vi "Import VeriStand Mappings.vi"() -> ()   [LabVIEW 2016]
uses:
  NationalInstruments.VeriStand.SystemDefinitionAPI
  <vilib>/Utility/file.llb/Read Delimited Spreadsheet (string).vi
panel:
  out "String":string="Running..."
  in  "System Definition File (.nivssdf)":path
  in  "System Mappings File (.txt)":path
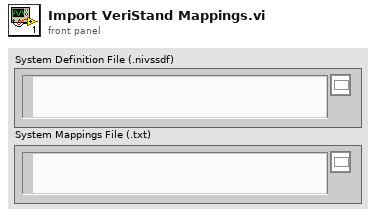
[diagram p1: front panel]
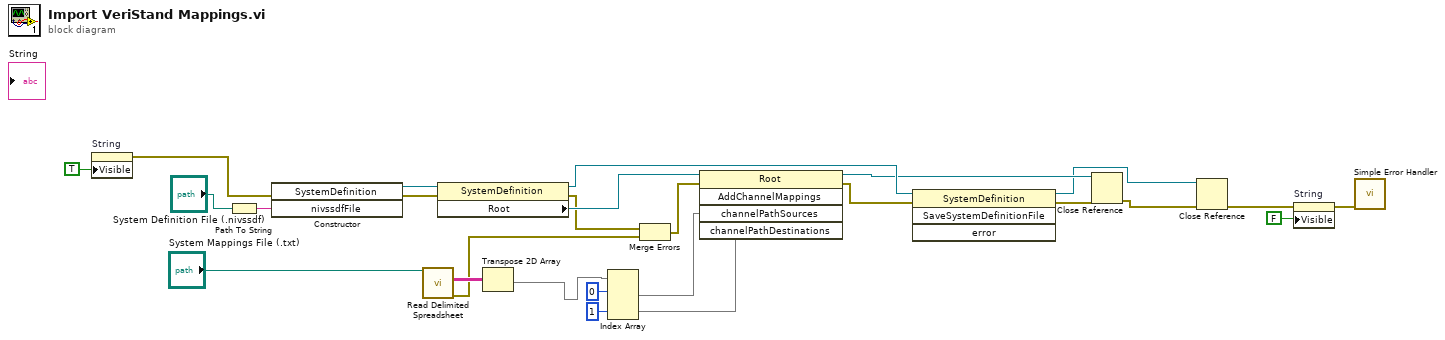
[diagram p0: block diagram]
diagram:
  n1 = property on="String" class="Str"("Visible"=TRUE) -> (error out=w4:errorcluster)  [unwired: 2 in, 1 out]
  n2 = Path To String(path="System Definition File (.nivssdf)") -> (string=w6:string)
  n3 = constructor class="SystemDefinition"(error in=w4, "nivssdfFile"=w6) -> (reference out=w25:refnum<k24>, error out=w21:errorcluster)  [unwired: 2 in, 2 out]
  n4 = call-poly <vilib>:"Read Delimited Spreadsheet.vi"("file path (dialog if empty)"="System Mappings File (.txt)") -> ("all rows"=w15:string[][], "error out"=w8:errorcluster)  [unwired: 9 in, 4 out]
  n5 = property class="SystemDefinition"(reference=w25, error in=w21) -> (reference out=w23:refnum<k24>, error out=w9:errorcluster, "Root"=w24:refnum<k24>)
  n6 = Transpose 2D Array(2D array=w15) -> (transposed array=w12:string[][])
  n7 = Index Array(array=w12, index (row) #1=0 ("index"), index (row) #2=1 ("index")) -> (element #1=w11:string[], element #2=w10:string[])  [unwired: 2 in]
  n8 = Merge Errors(w9, w8) -> (w7:errorcluster)
  n9 = invoke class="Root" method="AddChannelMappings"(reference=w24, error in=w7, "channelPathSources"=w11, "channelPathDestinations"=w10) -> (reference out=w20:refnum<k24>, error out=w22:errorcluster)  [unwired: 1 in, 3 out]
  n10 = invoke class="SystemDefinition" method="SaveSystemDefinitionFile"(reference=w23, error in=w22) -> (reference out=w17:refnum<k24>, error out=w19:errorcluster)  [unwired: 2 in, 2 out]
  n11 = Close Reference(reference=w20, error in (no error)=w19) -> (error out=w18:errorcluster)
  n12 = Close Reference(reference=w17, error in (no error)=w18) -> (error out=w2:errorcluster)
  n13 = property on="String" class="Str"(error in=w2, "Visible"=FALSE) -> (error out=w1:errorcluster)  [unwired: 1 in, 1 out]
  n14 = call <vilib>:"Simple Error Handler.vi"("error in (no error)"=w1) -> ()  [unwired: 4 in, 5 out]
